vi "Symphony Acquire Image.vi"(5 "Acquire":refnum<vi>, 7 "Running":refnum<vi>, 8 "Error In":errorcluster, 10 "ShutterOpen":bool, 11 "JYCCDLib.IJYCCDReqd":refnum<k7>) -> (0 "Acq Time(ms)":u32, 3 "Raw Data":i32[][][](array[numeric]))   [LabVIEW 2010]
panel:
  out "ReadyForAcquisition":bool
  out "AcquisitionBusy":bool
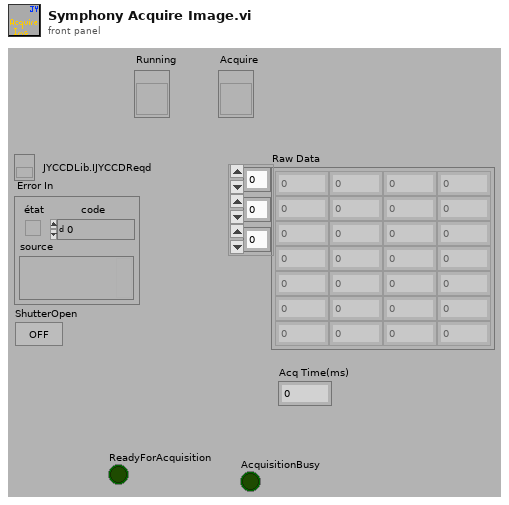
[diagram p1: front panel]
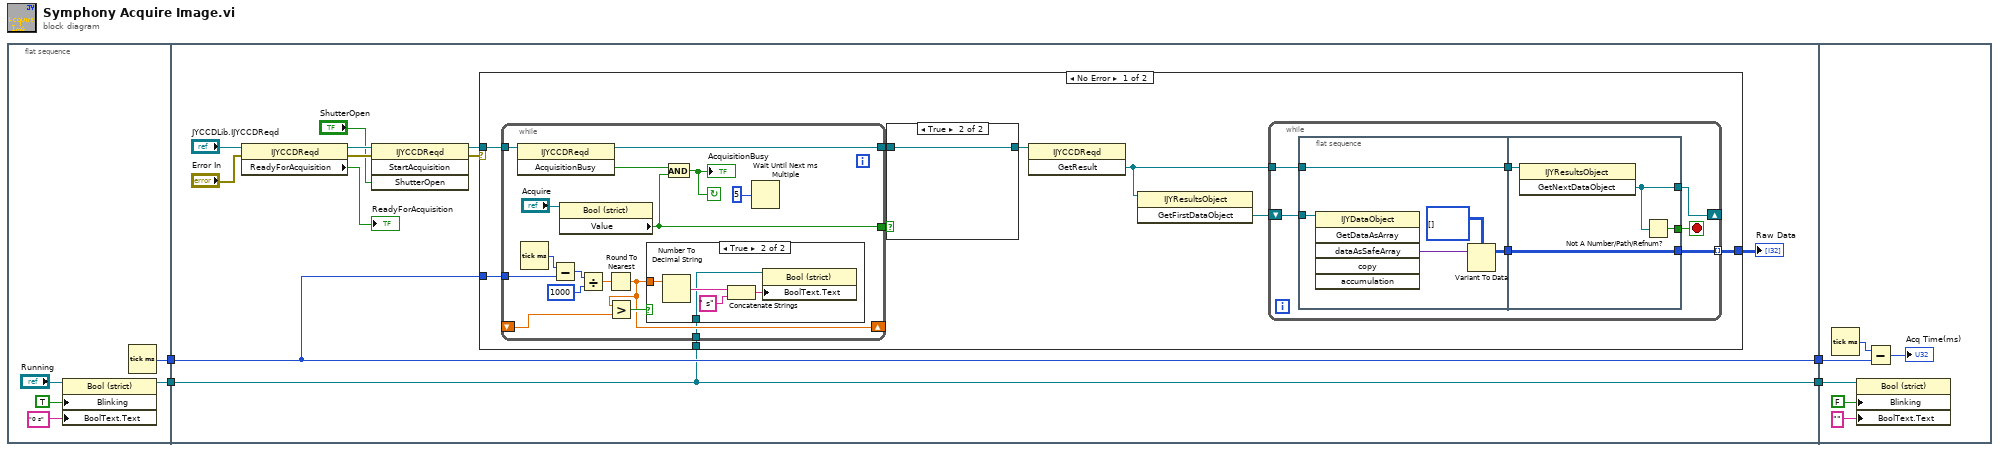
[diagram p0: block diagram]
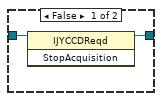
[diagram p2: hidden frame]
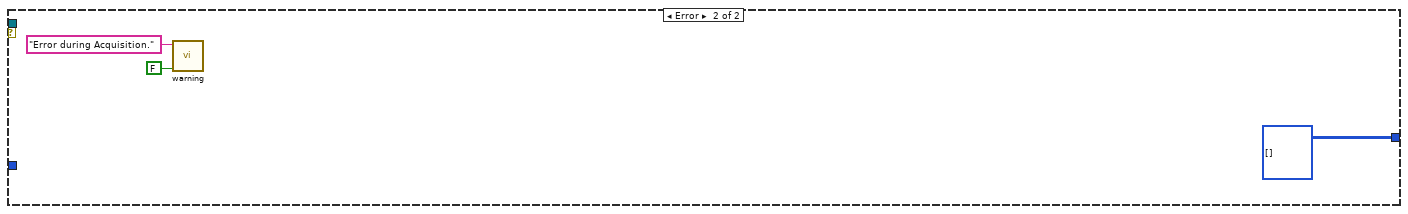
[diagram p4: hidden frame]
diagram:
  n1 = flat-sequence {
    tunnel: [w6] -> w3
    tunnel: [w5] -> w1
    tunnel: [w11] -> w4
    tunnel: w3 -> [w11]
    tunnel: [w10] -> w2
    tunnel: w1 -> [w10]
    tunnel: w4 -> [w74]
    tunnel: w2 -> [w73]
    frame #0 {
      n2 = property class="Bool (strict)"(reference="Running", "Blinking"=TRUE ("Blinkend"), "BoolText.Text"="0 s" ("Boolean Text.Text")) -> (reference out=w5:refnum<vi>)  [unwired: 1 in, 1 out]
      n3 = Tick Count (ms)() -> (millisecond timer value=w6:u32)
    }
    frame #1 {
      n4 = property class="IJYCCDReqd"(reference="JYCCDLib.IJYCCDReqd", error in="Error In") -> (reference out=w16:refnum<k7>, error out=w15:errorcluster, "ReadyForAcquisition"=→"ReadyForAcquisition":bool)
      n5 = invoke class="IJYCCDReqd" method="StartAcquisition"(reference=w16, error in=w15, "ShutterOpen"="ShutterOpen") -> (reference out=w20:refnum<k7>, error out=w19:errorcluster)  [unwired: 1 in, 2 out]
      n6 = case shown="No Error" w19 {
        tunnel: w20 -> [w29 _]
        tunnel: [w23 i32[][][] [] ("type")] -> w13
        tunnel: w11 -> [w22 _]
        tunnel: w10 -> [w21 _]
        frame No Error {
          n7 = while {
            tunnel: w29 -> [w64]
            tunnel: [w60] -> w25
            tunnel: [w58] -> w24
            tunnel: w22 -> [w52]
            shift-right: [w51] -> _
            shift-left: _ -> [w50]
            tunnel: w21 -> [w49]
            stop <- w59 continue-if-true
            n8 = invoke class="IJYCCDReqd" method="AcquisitionBusy"(reference=w64) -> (reference out=w58:refnum<k7>, "AcquisitionBusy"=w61:bool)  [unwired: 2 in, 1 out]
            n9 = Tick Count (ms)() -> (millisecond timer value=w56:u32)
            n10 = Subtract(x=w56, y=w52) -> (x-y=w55:u32)
            n11 = property class="Bool (strict)"(reference="Acquire") -> ("Value"=w60:bool)  [unwired: 1 in, 2 out]
            n12 = Divide(x=w55, y=u32 1000) -> (x/y=w57:dbl)
            n13 = Round To Nearest(number=w57) -> (nearest integer value=w51:dbl)
            n14 = Greater?(x=w51, y=w50) -> (0:w53:bool)
            n15 = case shown="True" w53 {
              tunnel: w51 -> [_ w69]
              tunnel: w49 -> [_ w65]
              frame False {
              }
              frame True {
                n16 = Number To Decimal String(number=w69) -> (decimal integer string=w68:string)  [unwired: 1 in]
                n17 = Concatenate Strings(w68, " s" ("string")) -> (w66:string)
                n18 = property class="Bool (strict)"(reference=w65, "BoolText.Text"=w66) -> ()  [unwired: 1 in, 2 out]
              }
            }
            n19 = And(x=w61, y=w60) -> (x .and. y?=w59:bool)
            "AcquisitionBusy" <- w59
            n20 = Wait Until Next ms Multiple(millisecond multiple=u32 5 ("n millisecondes")) -> ()  [unwired: 1 out]
          }
          n21 = case shown="True" w25 {
            tunnel: w24 -> [w47 w48]
            tunnel: [w46 w48] -> w26
            frame False {
              n22 = invoke class="IJYCCDReqd" method="StopAcquisition"(reference=w47) -> (reference out=w46:refnum<k7>)  [unwired: 2 in, 2 out]
            }
            frame True {
            }
          }
          n23 = invoke class="IJYCCDReqd" method="GetResult"(reference=w26) -> ("GetResult"=w27:refnum<k7>)  [unwired: 2 in, 2 out]
          n24 = invoke class="IJYResultsObject" method="GetFirstDataObject"(reference=w27) -> ("GetFirstDataObject"=w28:refnum<k7>)  [unwired: 2 in, 2 out]
          n25 = while {
            tunnel: [w33] -> w23 mode=indexing
            tunnel: w27 -> [w35]
            shift-left: w28 -> [w36]
            shift-right: [w34] -> _
            stop <- w32 stop-if-true
            n26 = flat-sequence {
              tunnel: w36 -> [w39]
              tunnel: w35 -> [w37]
              tunnel: [w37] -> w31
              tunnel: [w38] -> w30
              tunnel: w31 -> [w45]
              tunnel: [w44] -> w34
              tunnel: [w42] -> w33
              tunnel: w30 -> [w42]
              tunnel: [w43] -> w32
              frame #0 {
                n27 = invoke class="IJYDataObject" method="GetDataAsArray"(reference=w39) -> ("dataAsSafeArray"=w40:variant)  [unwired: 5 in, 5 out]
                n28 = Variant To Data(Variant=w40, type=i32[][] []) -> (data=w38:i32[][])  [unwired: 1 in, 1 out]
              }
              frame #1 {
                n29 = invoke class="IJYResultsObject" method="GetNextDataObject"(reference=w45) -> ("GetNextDataObject"=w44:refnum<k7>)  [unwired: 2 in, 2 out]
                n30 = Not A Number/Path/Refnum?(number/path/refnum=w44) -> (NaN/Path/Refnum?=w43:bool)
              }
            }
          }
        }
        frame Error {
          n31 = call "warning.vi"("with cancel ?"=FALSE, "Text"="Error during Acquisition.") -> ()  [unwired: 2 in, 1 out]
        }
      }
      "Raw Data" <- w13
    }
    frame #2 {
      n32 = Tick Count (ms)() -> (millisecond timer value=w75:u32)
      n33 = property class="Bool (strict)"(reference=w73, "Blinking"=FALSE ("Blinkend"), "BoolText.Text"="" ("Boolean Text.Text")) -> ()  [unwired: 1 in, 2 out]
      n34 = Subtract(x=w75, y=w74) -> (x-y=→"Acq Time(ms)":u32)
    }
  }
